vi "Process Configuration Errors.vi"(6 "IED Name":string, 8 "error in (no error)":errorcluster) -> (0 "error out":errorcluster, 1 "Error String":string, 2 "Status":T1)   [LabVIEW 2015, in "IED Actor.lvlib" / "IED.lvclass"]
uses:
  IED.lvclass
  SCADA Core/SCADA Abstract Messages/Device Load Status Msg/Device Load Status.ctl
  <vilib>/Utility/error.llb/DialogType.ctl
  SCADA Core/SCADA Abstract Messages/Device Load Status Msg/Device Load Status Msg.lvclass
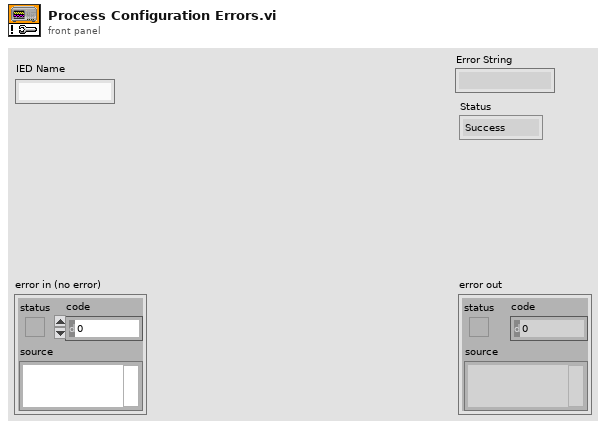
[diagram p1: front panel]
types:
  T1 = typedef "SCADA Core.lvlib/Device Load Status Msg.lvclass/Device Load Status.ctl" = enum16{"Success", "Failure"}
  T2 = typedef "DialogType.ctl" = u16
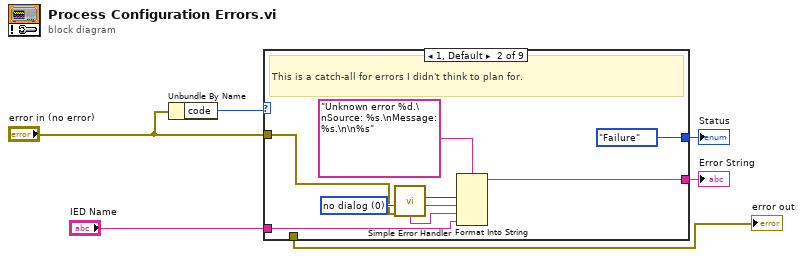
[diagram p0: block diagram]
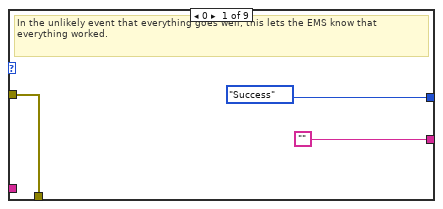
[diagram p2: hidden frame]
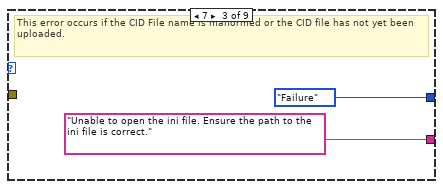
[diagram p3: hidden frame]
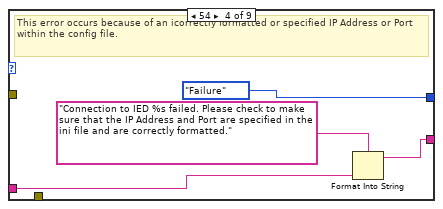
[diagram p4: hidden frame]
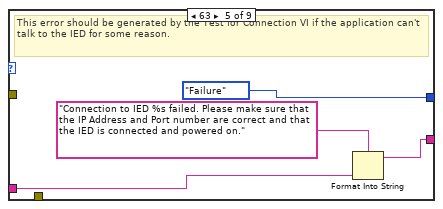
[diagram p5: hidden frame]
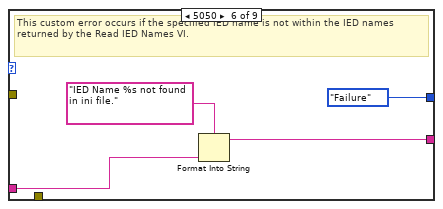
[diagram p6: hidden frame]
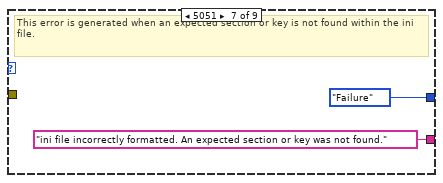
[diagram p7: hidden frame]
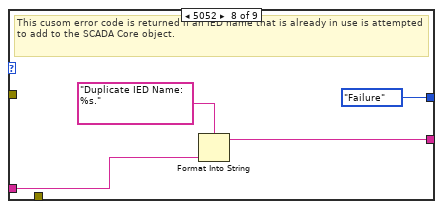
[diagram p8: hidden frame]
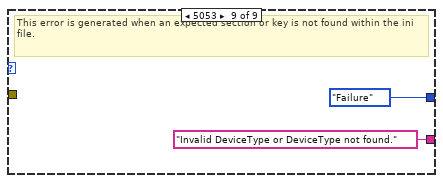
[diagram p9: hidden frame]
diagram:
  n1 = Unbundle By Name("error in (no error)") -> ("code"=w5:i32)
  n2 = case shown="1, Default" w5 {
    tunnel: [Device_Load_Status."Success" ("Status") Device_Load_Status."Failure" ("Status") Device_Load_Status."Failure" ("Status") Device_Load_Status."Failure" ("Status") Device_Load_Status."Failure" ("Status") Device_Load_Status."Failure" ("Status") Device_Load_Status."Failure" ("Status") Device_Load_Status."Failure" ("Status") Device_Load_Status."Failure" ("Status")] -> w4
    tunnel: ["" w13 "Unable to open the ini file. Ensure the path to the ini file is correct." ("Error String") w21 w25 w31 "ini file incorrectly formatted. An expected section or key was not found." ("Error String") w37 "Invalid DeviceType or DeviceType not found." ("Error String")] -> w3
    tunnel: "error in (no error)" -> [w8 w12 _ _ _ _ _ _ _]
    tunnel: [w8 _ _ _ _ _ _ _ _] -> w2
    tunnel: "IED Name" -> [_ w11 _ w22 w26 w30 _ w36 _]
    frame 0 {
      # "In the unlikely event that everything goes well, this lets the EMS know that everything worked."
    }
    frame 1, Default {
      w18 = T2 0 items=["no dialog", "OK message", "continue or stop message", "OK message + warnings", "continue/stop + warnings"] ("type of dialog (OK msg:1)")
      # "This is a catch-all for errors I didn't think to plan for."
      n3 = call <vilib>:"Simple Error Handler.vi"("type of dialog (OK msg:1)"=w18, "error in (no error)"=w12) -> ("code out"=w16:i32, "source out"=w15:string, "message"=w14:string)  [unwired: 3 in, 2 out]
      n4 = Format Into String(format string="Unknown error %d.\nSource: %s.\nMessage: %s.\n\n%s" ("Error String"), w16, w15, w14, w11) -> (resulting string=w13:string)  [unwired: 2 in, 1 out]
    }
    frame 7 {
      # "This error occurs if the CID File name is malformed or the CID file has not yet been uploaded."
    }
    frame 54 {
      # "This error occurs because of an icorrectly formatted or specified IP Address or Port within the config file."
      n5 = Format Into String(format string="Connection to IED %s failed. Please check to make sure that the IP Address and Port are specified in the ini file and are correctly formatted." ("Error String"), w22) -> (resulting string=w21:string)  [unwired: 2 in, 1 out]
    }
    frame 63 {
      # "This error should be generated by the Test for Connection VI if the application can't talk to the IED for some reason."
      n6 = Format Into String(format string="Connection to IED %s failed. Please make sure that the IP Address and Port number are correct and that the IED is connected and powered on." ("Error String"), w26) -> (resulting string=w25:string)  [unwired: 2 in, 1 out]
    }
    frame 5050 {
      # "This custom error occurs if the specified IED name is not within the IED names returned by the Read IED Names VI."
      n7 = Format Into String(format string="IED Name %s not found in ini file." ("Error String"), w30) -> (resulting string=w31:string)  [unwired: 2 in, 1 out]
    }
    frame 5051 {
      # "This error is generated when an expected section or key is not found within the ini file."
    }
    frame 5052 {
      # "This cusom error code is returned if an IED name that is already in use is attempted to add to the SCADA Core object."
      n8 = Format Into String(format string="Duplicate IED Name: %s." ("Error String"), w36) -> (resulting string=w37:string)  [unwired: 2 in, 1 out]
    }
    frame 5053 {
      # "This error is generated when an expected section or key is not found within the ini file."
    }
  }
  "error out" <- w2
  "Status" <- w4
  "Error String" <- w3
